vi "Read Position Props.vi"(8 "error in (no error)":errorcluster, 11 "Ctl Refnum in":refnum<vi>) -> (0 "error out":errorcluster, 2 "Position Props":T1, 3 "Ctl Refnum":refnum<vi>)   [LabVIEW 2020, in "VolatusGUIEditorCore.lvlib"]
uses:
  VolatusGUIEditorCore.lvlib
  Position Props.ctl
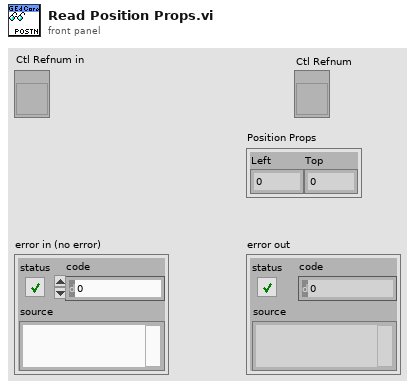
[diagram p1: front panel]
types:
  T1 = typedef "VolatusGUIEditorCore.lvlib/Position Props.ctl" = cluster{"Left":i32, "Top":i32}
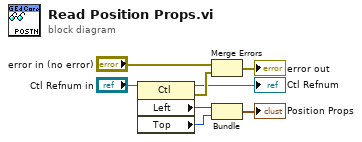
[diagram p0: block diagram]
diagram:
  n1 = property class="Ctl"(reference="Ctl Refnum in") -> (reference out=→"Ctl Refnum":refnum<vi>, error out=w6:errorcluster, "Left"=w3:i32, "Top"=w2:i32)  [unwired: 1 in]
  n2 = Merge Errors("error in (no error)", w6) -> (→"error out":errorcluster)
  n3 = Bundle("Left"=w3, "Top"=w2) -> (→"Position Props":cluster{"Left":i32, "Top":i32})  [unwired: 1 in]
